vi "Encode Parameters into Words for Labels in a Channel.vi"(7 "reset index":bool, 8 "error in (no error)":errorcluster, 9 "labels settings for RT in":T2[](array[typedef]) {"Label Timestamp Channel Data Reference" format="%.0x"; "Word Initial Raw Value" format="%032.0f"; "Label Disable/Trigger Channel Reference" format="%.0x"; "parameter driver data"."Tx parameter refs" format="%.0x"; "SDI" format="%02b"; "label" format="%.0o"}, 10 "Triggers in":bool[](array[boolean]), 11 "Parameter Values in":dbl[](array[numeric])) -> (0 "error out":errorcluster, 2 "data with triggers out":T1[](array[typedef]))   [LabVIEW 2020, in "AIM ARINC 429 Engine.lvlib" / "Implementation.lvlib" / "Tx Acyclic Labels Execution Unit.lvclass"]
uses:
  Tx Acyclic Labels Execution Unit.lvclass
  Shared/RT Label Settings.ctl
  Shared/Label.ctl
  Shared/RT Parameters.ctl
  Shared/Parameter Definition.ctl
  <vilib>/NI/NI VeriStand Encoding and Decoding/Encoding.ctl
  <vilib>/NI VeriStand/Custom Device API/Custom Device Item Ref.ctl
  Shared/Transfer Type.ctl
  <vilib>/NI VeriStand/Custom Device API/Data Reference.ctl
  Hardware API/Data Word with Trigger.ctl
  Shared/Encode Parameter and Update Word (32-bit).vi/1445f95d-237d-4fc6-96b9-8992d347f513.vi
  Shared/Encode Parameter and Update Word (32-bit).vi/6b8853f0-8e5d-49e3-9391-4d3f8e5314b0.vi
  Shared/Encode Parameter and Update Word (32-bit).vi/2babc4f4-546e-4d35-846d-a4a1fbac0249.vi
  Shared/Encode Parameter and Update Word (32-bit).vi/1445f95d-237d-4fc6-96b9-8992d347f513.vi/9377bb8f-44b5-4a8f-87f1-966fd5a9edcc.vi
  Shared/Encode Parameter and Update Word (32-bit).vi/1445f95d-237d-4fc6-96b9-8992d347f513.vi/e95d9d1f-307c-44d6-9f26-c3f519a4990d.vi
  Shared/Encode Parameter and Update Word (32-bit).vi/1445f95d-237d-4fc6-96b9-8992d347f513.vi/0c23f515-4369-4514-bc3d-4444e6b437b2.vi
  Shared/Encode Parameter and Update Word (32-bit).vi/6b8853f0-8e5d-49e3-9391-4d3f8e5314b0.vi/136dcdcb-2dd3-4a4d-a796-a8f7a3f8e1ac.vi
  Shared/Encode Parameter and Update Word (32-bit).vi/6b8853f0-8e5d-49e3-9391-4d3f8e5314b0.vi/a54b505c-1216-4ef4-8378-3ceda9d188df.vi
  <vilib>/NI/NI VeriStand Encoding and Decoding/Get Bits Per Digit from Base.vi
  Hardware API/AIM ARINC 429 Hardware API.lvlib
  <vilib>/NI/NI VeriStand Encoding and Decoding/Encoding and Decoding.lvlib
  <vilib>/NI VeriStand/Custom Device API/Custom Device API.lvlib
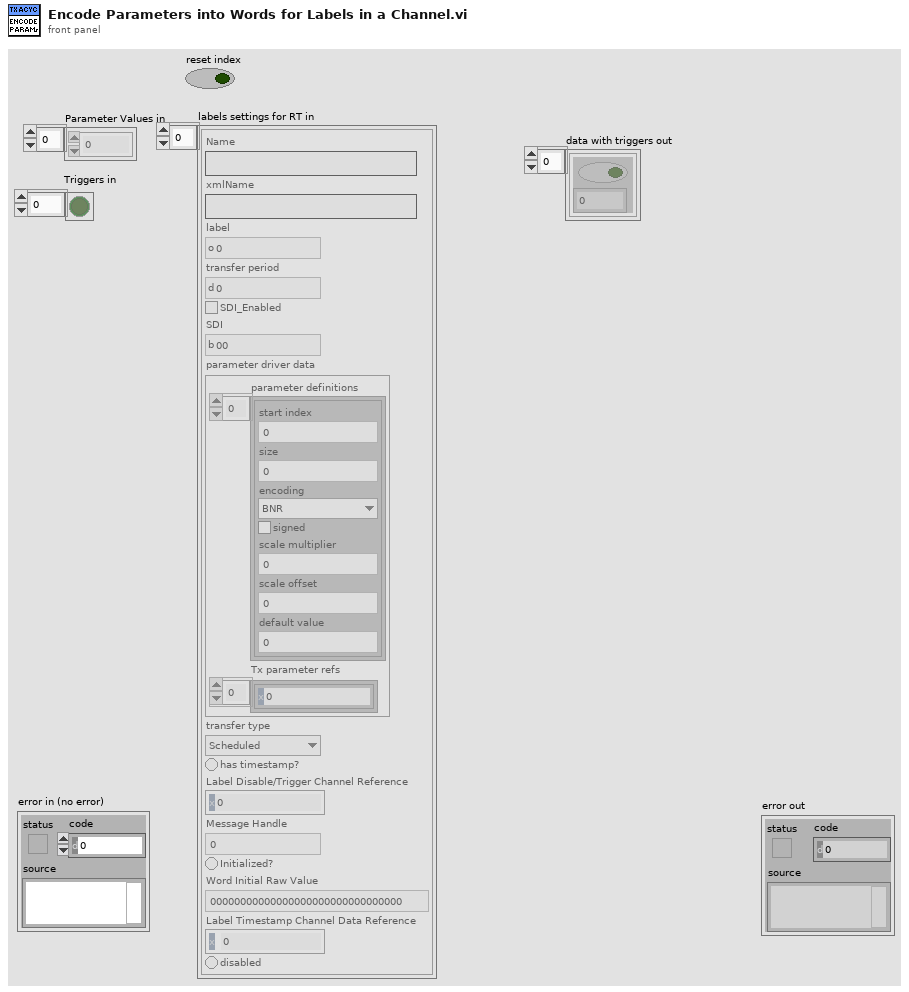
[diagram p1: front panel]
types:
  T1 = typedef "AIM ARINC 429 Hardware API.lvlib/Data Word with Trigger.ctl" = cluster{"Trigger":bool, "Data Word":u32}
  T2 = typedef "RT Label Settings.ctl" = cluster{"Name":string, "xmlName":string, "label":T3, "transfer period":u32, "SDI_Enabled":bool, "SDI":u8, "parameter driver data":T4, "transfer type":T8, "has timestamp?":bool, "Label Disable/Trigger Channel Reference":T7, "Message Handle":u64, "Initialized?":bool, "Word Initial Raw Value":u32, "Label Timestamp Channel Data Reference":T9, "disabled":bool}
  T3 = typedef "Label.ctl" = u8
  T4 = typedef "RT Parameters.ctl" = cluster{"parameter definitions":T5[], "Tx parameter refs":T7[]}
  T5 = typedef "Parameter Definition.ctl" = cluster{"start index":i32, "size":i32, "encoding":T6, "signed":bool, "scale multiplier":dbl, "scale offset":dbl, "default value":dbl}
  T6 = typedef "Encoding and Decoding.lvlib/Encoding.ctl" = enum16{"BNR", "BCD", "Discrete"}
  T7 = typedef "Custom Device API.lvlib/Custom Device Item Ref.ctl" = u64
  T8 = typedef "Transfer Type.ctl" = enum16{"Scheduled", "Acyclic", "Block", "Strobe"}
  T9 = typedef "Custom Device API.lvlib/Data Reference.ctl" = i32
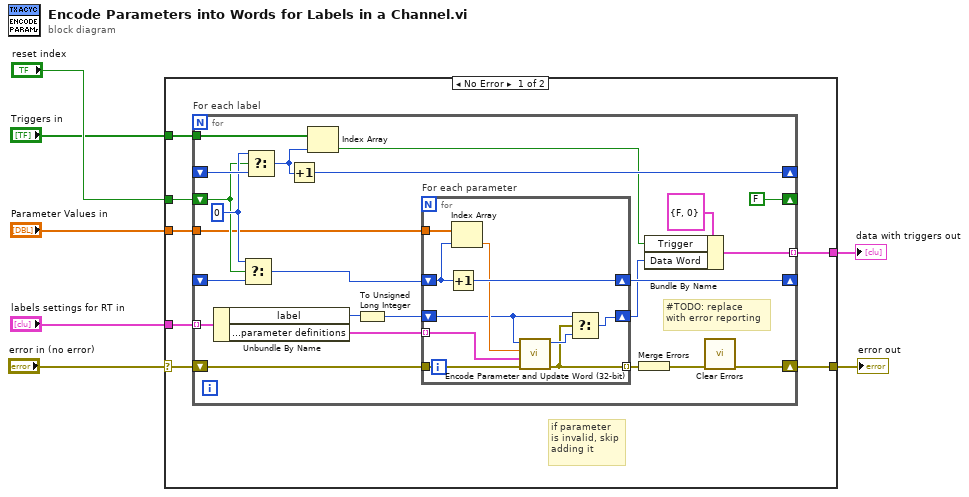
[diagram p0: block diagram]
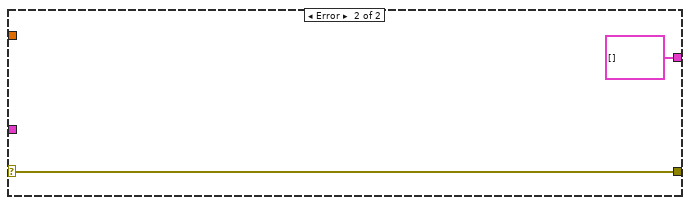
[diagram p2: hidden frame]
diagram:
  n1 = case shown="No Error" "error in (no error)" {
    selector: "error in (no error)" -> [w8 w48]
    tunnel: "reset index" -> [w14 _]
    tunnel: "Triggers in" -> [w13 _]
    tunnel: "Parameter Values in" -> [w12 _]
    tunnel: "labels settings for RT in" -> [w11 _]
    tunnel: [w10 w48] -> w3
    tunnel: [w9 T1[] []] -> w2
    frame No Error {
      # "if parameter\nis invalid, skip\nadding it"
      n2 = for "For each label" {
        shift-right: [FALSE ("reset index")] -> _
        shift-left: w14 -> [w25]
        tunnel: w13 -> [w24]
        tunnel: w12 -> [w21]
        tunnel: w11 -> [w35] mode=indexing
        shift-right: [w15] -> w10
        shift-left: w8 -> [w37]
        shift-right: [w29] -> _
        shift-left: _ -> [w31]
        shift-right: [w22] -> _
        shift-left: _ -> [w27]
        tunnel: [w17] -> w9 mode=indexing
        w26 = 0 ("index")
        # "#TODO: replace\nwith error reporting"
        n3 = Unbundle By Name(w35) -> ("label"=w34:T3, "parameter driver data.parameter definitions"=w32:T5[])
        n4 = Select(t=w26, s=w25, f=w31) -> (s? t:f=w30:i32)
        n5 = Select(t=w26, s=w25, f=w27) -> (s? t:f=w23:i32)
        n6 = Increment(x=w23) -> (x+1=w22:i32)
        n7 = Index Array(array=w24, index=w23) -> (element=w19:bool)
        n8 = To Unsigned Long Integer(number=w34) -> (unsigned 32bit integer=w33:u32)
        n9 = for "For each parameter" {
          shift-right: [w41] -> w18
          shift-left: w33 -> [w39]
          tunnel: w32 -> [w46] mode=indexing
          shift-right: [w43] -> w29
          shift-left: w30 -> [w44]
          tunnel: w21 -> [w45]
          tunnel: w37 -> [w47]
          tunnel: [w38] -> w36 mode=indexing
          n10 = Increment(x=w44) -> (x+1=w43:i32)
          n11 = Index Array(array=w45, index=w44) -> (element=w42:dbl)
          n12 = call "Encode Parameter and Update Word (32-bit).vi"("error in"=w47, "parameter definition"=w46, "parameter value"=w42, "word in"=w39) -> ("error out"=w38:errorcluster, "word out"=w40:u32)  [unwired: 6 in]
          n13 = Select(t=w39, s=w38, f=w40) -> (s? t:f=w41:u32)
        }
        n14 = Merge Errors(w36) -> (w16:errorcluster)
        n15 = Bundle By Name(cluster=T1 {"Trigger"=FALSE, "Data Word"=0} ("Word with Trigger"), "Trigger"=w19, "Data Word"=w18) -> (w17:T1)
        n16 = call <vilib>:"Clear Errors.vi"("error in (no error)"=w16) -> ("error out"=w15:errorcluster)  [unwired: 5 in, 1 out]
      }
    }
    frame Error {
    }
  }
  "error out" <- w3
  "data with triggers out" <- w2
